vi "FormIO.vi"() -> ()   [LabVIEW 2012]
uses:
  S7Ref.vi
  resultShow.vi
panel:
  in  "数值 3":dbl format="%#_4g"
  in  "布尔":bool
  out "DI 4":T1
  out "DI 5":T1
  in  "DQ 4":T1
  in  "DQ 5":T1
  in  "DQ 6":T2
  in  "选项卡控件":enum32{"开关信号/操作", "传感器信号"}(tab)
  out "DI 0":T3
  out "DI 2":T4
  out "DI 1":T5
  out "DI 3":T6
  in  "DQ 0":T7
  in  "DQ 1":T8
  in  "DQ 2":T9
  in  "DQ 3":T1
  in  "数值 2":dbl format="%#_4g"
  out "AI":T11 {"V    AI 7" format="%#.2g"; "V    AI 6" format="%#.2g"; "V    AI 5" format="%#.2g"; "V    AI 4" format="%#.2g"; "V    AI 3" format="%#.2g"; "V    AI 2" format="%#.2g"; "V    AI 1" format="%#.2f"; "N/m 扭矩传感器" format="%#.2g"}
  in  "校准":bool
  # "输入上"
  # "输入下"
  # "输出上"
  # "输出下"
  # "输入正"
  # "输入反"
  # "输出正"
  # "输出反"
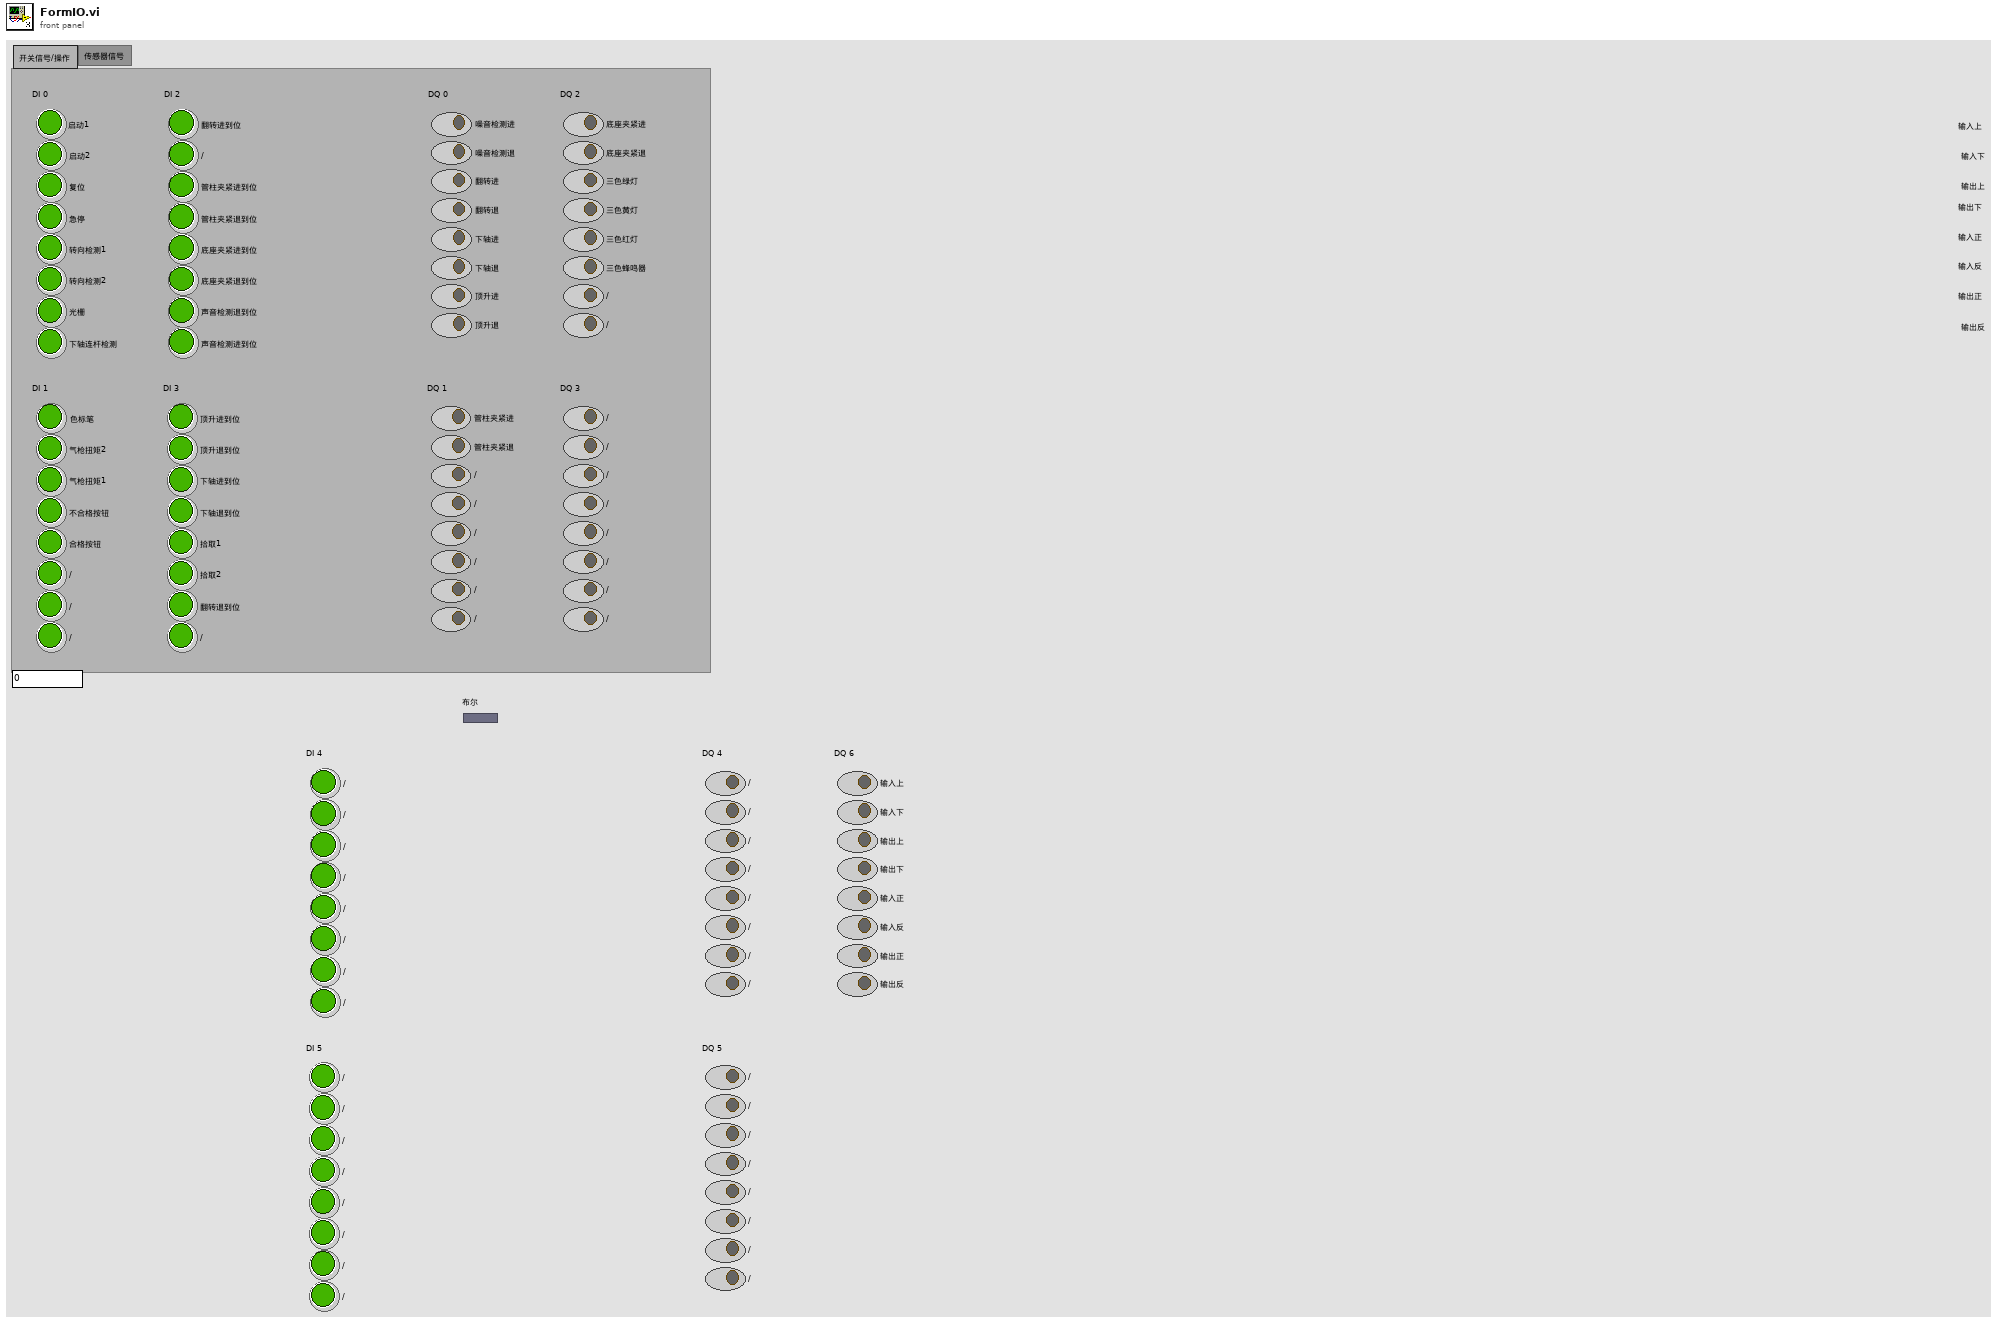
[diagram p1: front panel]
types:
  T1 = cluster{"/":bool, "/":bool, "/":bool, "/":bool, "/":bool, "/":bool, "/":bool, "/":bool}
  T2 = cluster{"输入上":bool, "输入下":bool, "输出上":bool, "输出下":bool, "输入正":bool, "输入反":bool, "输出正":bool, "输出反":bool}
  T3 = cluster{"启动1":bool, "启动2":bool, "复位":bool, "急停":bool, "转向检测1":bool, "转向检测2":bool, "光栅":bool, "下轴连杆检测":bool}
  T4 = cluster{"翻转进到位":bool, "/":bool, "管柱夹紧进到位":bool, "管柱夹紧退到位":bool, "底座夹紧进到位":bool, "底座夹紧退到位":bool, "声音检测退到位":bool, "声音检测进到位":bool}
  T5 = cluster{"色标笔":bool, "气枪扭矩2":bool, "气枪扭矩1":bool, "不合格按钮":bool, "合格按钮":bool, "/":bool, "/":bool, "/":bool}
  T6 = cluster{"顶升进到位":bool, "顶升退到位":bool, "下轴进到位":bool, "下轴退到位":bool, "拾取1":bool, "拾取2":bool, "翻转退到位":bool, "/":bool}
  T7 = cluster{"噪音检测进":bool, "噪音检测退":bool, "翻转进":bool, "翻转退":bool, "下轴进":bool, "下轴退":bool, "顶升进":bool, "顶升退":bool}
  T8 = cluster{"管柱夹紧进":bool, "管柱夹紧退":bool, "/":bool, "/":bool, "/":bool, "/":bool, "/":bool, "/":bool}
  T9 = cluster{"底座夹紧进":bool, "底座夹紧退":bool, "三色绿灯":bool, "三色黄灯":bool, "三色红灯":bool, "三色蜂鸣器":bool, "/":bool, "/":bool}
  T10 = typedef "控件 1.ctl" = dbl
  T11 = cluster{"N/m 扭矩传感器":dbl, "V    AI 1":T10, "V    AI 2":dbl, "V    AI 3":dbl, "V    AI 4":dbl, "V    AI 5":dbl, "V    AI 6":dbl, "V    AI 7":dbl}
  T12 = cluster{"输入移正脉冲":bool, "输入移反脉冲":bool, "输出移正脉冲":bool, "输出移反脉冲":bool, "控制器转速":bool, "/":bool, "控制器车速":bool, "/":bool}
  T13 = cluster{bool, bool, bool, bool, bool, bool, bool, bool}
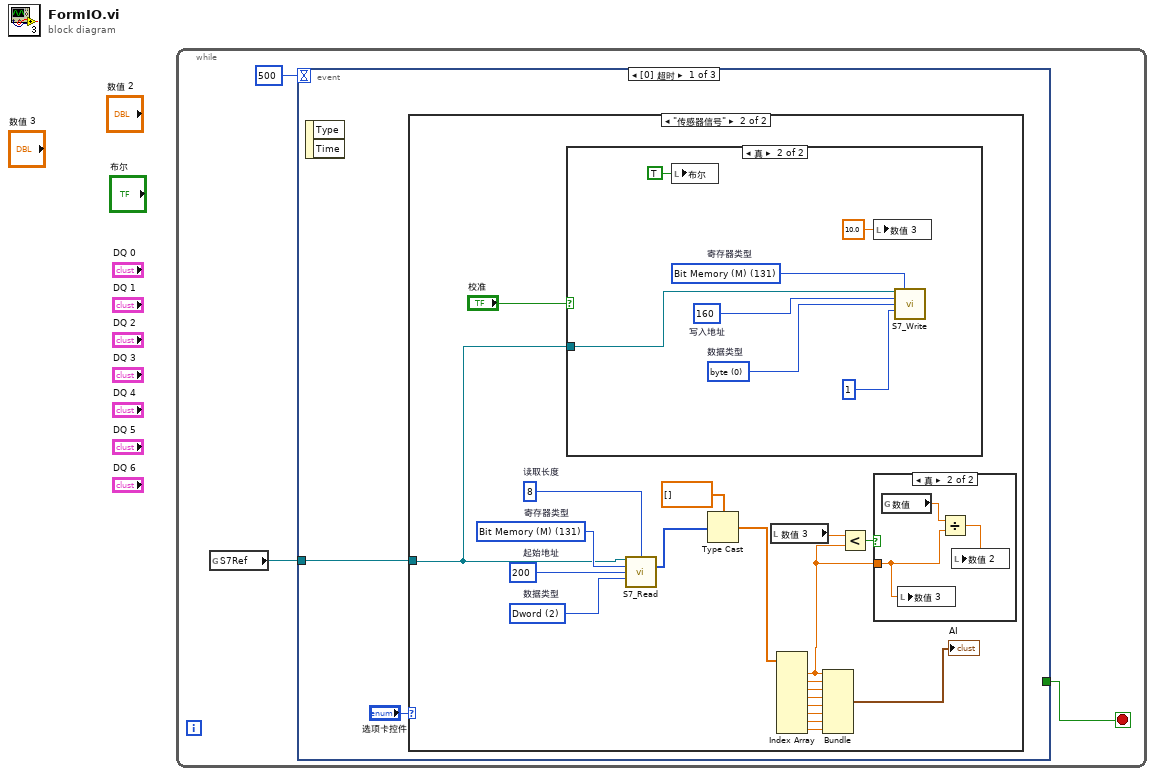
[diagram p0: block diagram]
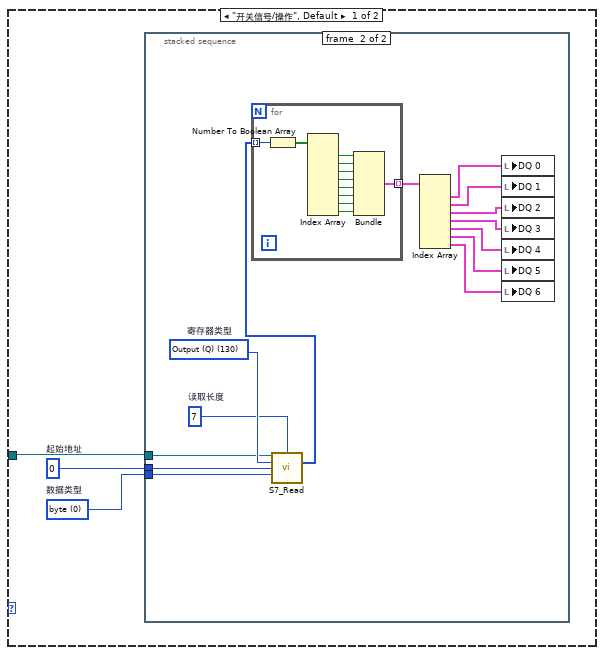
[diagram p2: hidden frame]
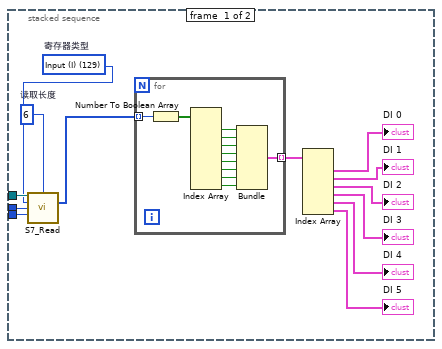
[diagram p3: hidden frame]
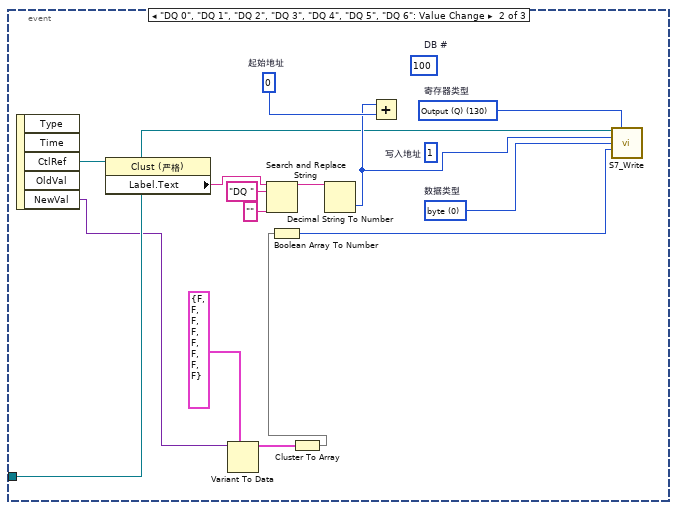
[diagram p6: hidden frame]
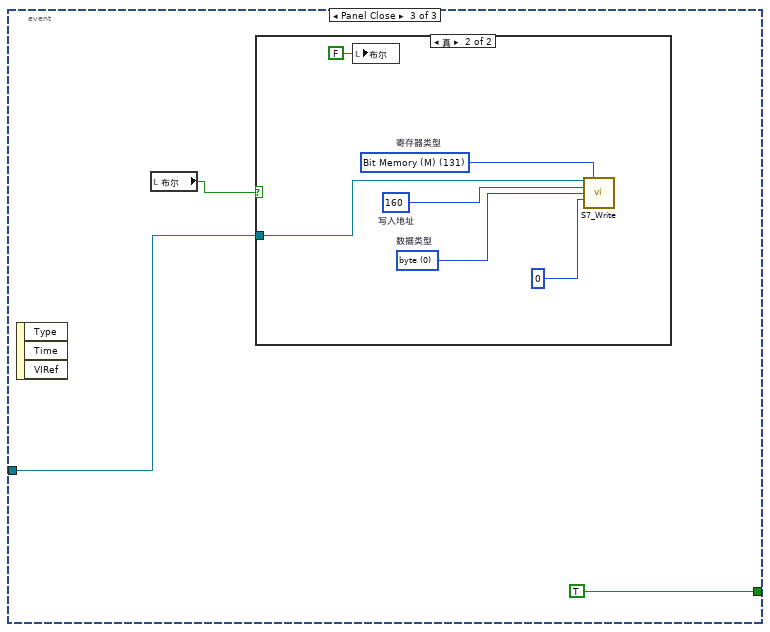
[diagram p7: hidden frame]
diagram:
  n1 = while {
    stop <- w3 stop-if-true
    n2 = global read "S7Ref.vi" "S7Ref"() -> (w1:refnum<k5>)
    n3 = event shown="[0] 超时" {
      selector: _ -> [_ _ _]
      dyn-events: _ -> [_ _ _]
      timeout: 500 -> [_ _ _]
      tunnel: [_ _ TRUE ("布尔")] -> w3
      tunnel: w1 -> [w4 w96 w104]
      event Timeout {
        n4 = event-data() -> ()  [unwired: 1 in, 2 out]
        n5 = case shown="\"传感器信号\"" "选项卡控件" {
          tunnel: w4 -> [w8 w62]
          frame "开关信号/操作", Default {
            w6 = u16 0 items=["byte", "word", "Dword"]  # 数据类型
            w7 = u32 0  # 起始地址
            n6 = stacked-sequence {
              tunnel: w8 -> [w21 w45]
              tunnel: w7 -> [w20 w44]
              tunnel: w6 -> [w19 w43]
              frame #0 {
                w9 = u16 6  # 读取长度
                w18 = u8 129 items=["I/O (P)"=128, "Input (I)"=129, "Output (Q)"=130, "Bit Memory (M)"=131, "Data (DB)"=132, "Instance Data (DI)"=133, "Local Data (L)"=134, "Predecessor Local Data (VL)"=135]  # 寄存器类型
                n7 = call "S7_Read.vi"("TCP"=w21, "读取长度"=w9, "寄存器类型"=w18, "起始地址"=w20, "数据类型"=w19) -> ("数据"=w17:u32[])  [unwired: 7 in, 3 out]
                n8 = for {
                  tunnel: w17 -> [w32] mode=indexing
                  tunnel: [w22] -> w16 mode=indexing
                  n9 = Number To Boolean Array(number=w32) -> (Boolean array=w31:bool[])
                  n10 = Index Array(array=w31) -> (element #1=w30:bool, element #2=w29:bool, element #3=w28:bool, element #4=w27:bool, element #5=w26:bool, element #6=w25:bool, element #7=w24:bool, element #8=w23:bool)  [unwired: 8 in]
                  n11 = Bundle(w30, w29, w28, w27, w26, w25, w24, w23) -> (w22:T13)  [unwired: 1 in]
                }
                n12 = Index Array(array=w16) -> (element #1=→"DI 0":T13, element #2=→"DI 1":T13, element #3=→"DI 2":T13, element #4=→"DI 3":T13, element #5=→"DI 4":T13, element #6=→"DI 5":T13)  [unwired: 6 in]
              }
              frame #1 {
                w33 = u16 7  # 读取长度
                w46 = u8 130 items=["I/O (P)"=128, "Input (I)"=129, "Output (Q)"=130, "Bit Memory (M)"=131, "Data (DB)"=132, "Instance Data (DI)"=133, "Local Data (L)"=134, "Predecessor Local Data (VL)"=135]  # 寄存器类型
                n13 = call "S7_Read.vi"("TCP"=w45, "读取长度"=w33, "寄存器类型"=w46, "起始地址"=w44, "数据类型"=w43) -> ("数据"=w41:u32[])  [unwired: 7 in, 3 out]
                n14 = for {
                  tunnel: w41 -> [w57] mode=indexing
                  tunnel: [w47] -> w42 mode=indexing
                  n15 = Number To Boolean Array(number=w57) -> (Boolean array=w56:bool[])
                  n16 = Index Array(array=w56) -> (element #1=w55:bool, element #2=w54:bool, element #3=w53:bool, element #4=w52:bool, element #5=w51:bool, element #6=w50:bool, element #7=w49:bool, element #8=w48:bool)  [unwired: 8 in]
                  n17 = Bundle(w55, w54, w53, w52, w51, w50, w49, w48) -> (w47:T13)  [unwired: 1 in]
                }
                n18 = Index Array(array=w42) -> (element #1=w40:T13, element #2=w39:T13, element #3=w38:T13, element #4=w37:T13, element #5=w36:T13, element #6=w35:T13, element #7=w34:T13)  [unwired: 7 in]
                n19 = local write "DQ 0"(w40) -> ()
                n20 = local write "DQ 1"(w39) -> ()
                n21 = local write "DQ 2"(w38) -> ()
                n22 = local write "DQ 3"(w37) -> ()
                n23 = local write "DQ 4"(w36) -> ()
                n24 = local write "DQ 5"(w35) -> ()
                n25 = local write "DQ 6"(w34) -> ()
              }
            }
          }
          frame "传感器信号" {
            w75 = u16 2 items=["byte", "word", "Dword"]  # 数据类型
            w76 = u32 200  # 起始地址
            w77 = u8 131 items=["I/O (P)"=128, "Input (I)"=129, "Output (Q)"=130, "Bit Memory (M)"=131, "Data (DB)"=132, "Instance Data (DI)"=133, "Local Data (L)"=134, "Predecessor Local Data (VL)"=135]  # 寄存器类型
            w74 = u16 8  # 读取长度
            n26 = case shown="真" "校准" {
              tunnel: w62 -> [_ w87]
              frame False {
              }
              frame True {
                w84 = u16 0 items=["byte", "word", "Dword"]  # 数据类型
                w83 = u32 160  # 写入地址
                w85 = u8 131 items=["I/O (P)"=128, "Input (I)"=129, "Output (Q)"=130, "Bit Memory (M)"=131, "Data (DB)"=132, "Instance Data (DI)"=133, "Local Data (L)"=134, "Predecessor Local Data (VL)"=135]  # 寄存器类型
                n27 = local write "布尔"(TRUE ("布尔")) -> ()
                n28 = local write "数值 3"(10.0 ("数值 3")) -> ()
                n29 = call "S7_Write.vi"("TCP"=w87, "寄存器类型"=w85, "写入地址"=w83, "数据类型"=w84, "写入数据"=1) -> ()  [unwired: 8 in, 3 out]
              }
            }
            n30 = call "S7_Read.vi"("TCP"=w62, "读取长度"=w74, "寄存器类型"=w77, "起始地址"=w76, "数据类型"=w75) -> ("数据"=w72:u32[])  [unwired: 7 in, 3 out]
            n31 = Type Cast(type=sgl[] [] ("添加的数组"), x=w72) -> (*(type *) &x=w64:sgl[])
            n32 = local read "数值 3"() -> (w60:dbl)
            n33 = Index Array(array=w64) -> (element #1=w58:sgl, element #2=w65:sgl, element #3=w66:sgl, element #4=w67:sgl, element #5=w68:sgl, element #6=w69:sgl, element #7=w70:sgl, element #8=w71:sgl)  [unwired: 8 in]
            n34 = Bundle(w58, w65, w66, w67, w68, w69, w70, w71) -> (→"AI":cluster{sgl, sgl, sgl, sgl, sgl, sgl, sgl, sgl})  [unwired: 1 in]
            n35 = Less?(x=w60, y=w58) -> (x < y?=w59:bool)
            n36 = case shown="真" w59 {
              tunnel: w58 -> [_ w79]
              frame False {
              }
              frame True {
                n37 = global read "resultShow.vi" "数值"() -> (w80:dbl)
                n38 = local write "数值 3"(w79) -> ()
                n39 = Divide(x=w80, y=w79) -> (x/y=w78:dbl)
                n40 = local write "数值 2"(w78) -> ()
              }
            }
          }
        }
      }
      event "DQ 0", "DQ 1", "DQ 2", "DQ 3", "DQ 4", "DQ 5", "DQ 6": Value Change {
        w99 = u32 0  # 起始地址
        w101 = u16 0 items=["byte", "word", "Dword"]  # 数据类型
        (unwired) u32 1  # 写入地址
        (unwired) u16 100  # DB #
        w102 = u8 130 items=["I/O (P)"=128, "Input (I)"=129, "Output (Q)"=130, "Bit Memory (M)"=131, "Data (DB)"=132, "Instance Data (DI)"=133, "Local Data (L)"=134, "Predecessor Local Data (VL)"=135]  # 寄存器类型
        n41 = event-data() -> ("CtlRef"=w98:refnum<vi>, "NewVal"=w94:variant)  [unwired: 1 in, 3 out]
        n42 = property class="Clust (严格)"(reference=w98) -> ("Label.Text"=w89:string)  [unwired: 1 in, 2 out]
        n43 = Variant To Data(type=T12 {"输入移正脉冲"=FALSE, "输入移反脉冲"=FALSE, "输出移正脉冲"=FALSE, "输出移反脉冲"=FALSE, "控制器转速"=FALSE, "/"=FALSE, "控制器车速"=FALSE, "/"=FALSE} ("DQ 0"), Variant=w94) -> (data=w93:T12)  [unwired: 1 in, 1 out]
        n44 = Search and Replace String(input string=w89, search string="DQ " ("搜索字符串"), replace string="" ("替换字符串(\"\")")) -> (result string=w88:string)  [unwired: 5 in, 3 out]
        n45 = Cluster To Array(cluster=w93) -> (array=w92:bool[])
        n46 = Boolean Array To Number ("布尔数组至数值转换")(Boolean array=w92) -> (number=w100:u8)
        n47 = Decimal String To Number(string=w88) -> (number=w97:i32)  [unwired: 2 in, 1 out]
        n48 = Add(x=w97, y=w99) -> ()  [unwired: 1 out]
        n49 = call "S7_Write.vi"("TCP"=w96, "寄存器类型"=w102, "写入地址"=w97, "数据类型"=w101, "写入数据"=w100) -> ()  [unwired: 8 in, 3 out]
      }
      event Panel Close {
        n50 = event-data() -> ()  [unwired: 1 in, 3 out]
        n51 = local read "布尔"() -> (w103:bool)
        n52 = case shown="真" w103 {
          tunnel: w104 -> [_ w111]
          frame False {
          }
          frame True {
            w108 = u16 0 items=["byte", "word", "Dword"]  # 数据类型
            w107 = u32 160  # 写入地址
            w109 = u8 131 items=["I/O (P)"=128, "Input (I)"=129, "Output (Q)"=130, "Bit Memory (M)"=131, "Data (DB)"=132, "Instance Data (DI)"=133, "Local Data (L)"=134, "Predecessor Local Data (VL)"=135]  # 寄存器类型
            n53 = local write "布尔"(FALSE ("布尔")) -> ()
            n54 = call "S7_Write.vi"("TCP"=w111, "寄存器类型"=w109, "写入地址"=w107, "数据类型"=w108, "写入数据"=0) -> ()  [unwired: 8 in, 3 out]
          }
        }
      }
    }
  }
